vi "Assign Pixel to Wing Sector (FPGA).vi"(4 "End of Data?":bool, 6 "Valid Data?":bool, 7 "Pixel Intensity In":u8, 8 "Right Wing?":bool, 9 "Sector Parameters":T1, 10 "Pixel Y":u16, 11 "Pixel X":u16) -> (0 "Y Pixel Out":u16, 1 "Pixel Intensity Out":u8, 2 "sector #":u8, 3 "output valid":bool, 5 "X Pixel Out":u16)   [LabVIEW 2013]
uses:
  Sector Parameter Cluster.ctl
  <vilib>/rvi/FXPMathLib/FxpRectToPolar/subVIs/nifxpmath_RectToPolar_SimConfig.ctl
  <vilib>/rvi/FXPMathLib/FxpDiv/subVIs/nifxpmath_Div_SimConfig.ctl
  <vilib>/rvi/FXPMathLib/FxpRectToPolar/simVIs/DllFxpRectToPolarTemp_sub.vi
  <vilib>/rvi/FXPMathLib/FxpDiv/simVIs/DllFxpDivTemp_sub.vi
  <vilib>/rvi/FXPMathLib/FxpSub/XNode/nifxpmath_Sub.xnode
  <vilib>/rvi/FXPMathLib/FxpRectToPolar/XNode/nifxpmath_RectToPolar.xnode
  <vilib>/rvi/FXPMathLib/FxpAdd/XNode/nifxpmath_Add.xnode
  <vilib>/rvi/FXPMathLib/FxpDiv/XNode/nifxpmath_Div.xnode
  <vilib>/rvi/FXPMathLib/sim/FxpSim.dll
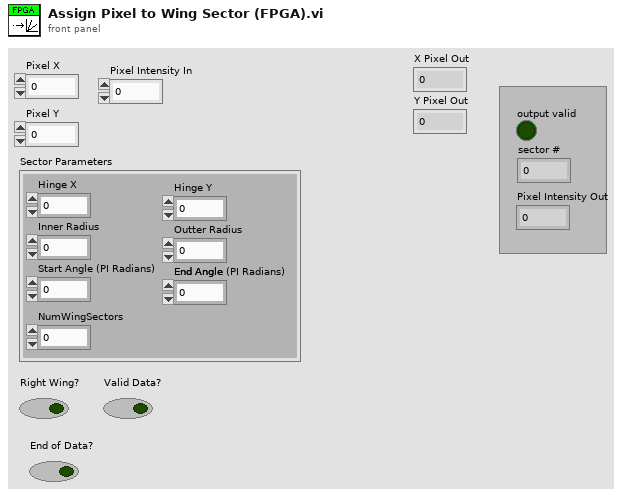
[diagram p1: front panel]
types:
  T1 = typedef "Sector Parameter Cluster.ctl" = cluster{"Start Angle":fxp<+/-,17,2>, "End Angle":fxp<+,17,3>, "Inner Radius":u16, "Outter Radius":u16, "Hinge X":u16, "Hinge Y":u16, "NumWingSectors":u8}
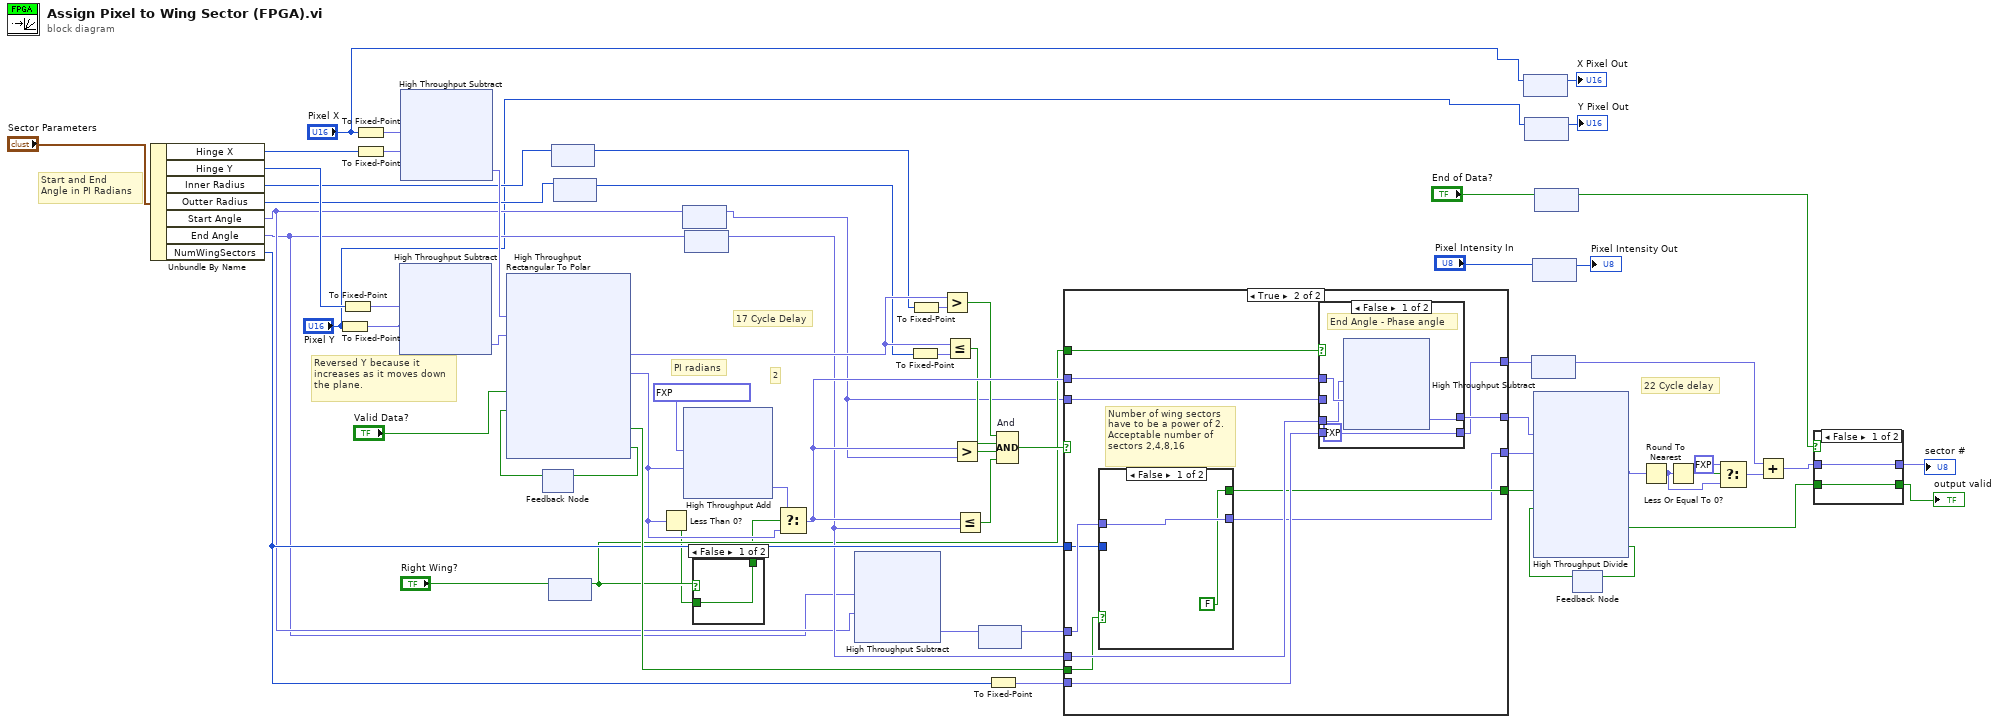
[diagram p0: block diagram]
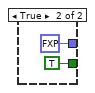
[diagram p2: hidden frame]
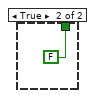
[diagram p3: hidden frame]
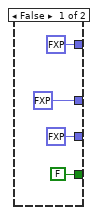
[diagram p4: hidden frame]
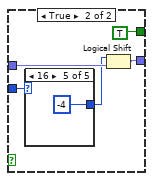
[diagram p5: hidden frame]
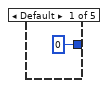
[diagram p6: hidden frame]
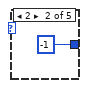
[diagram p7: hidden frame]
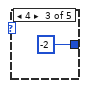
[diagram p8: hidden frame]
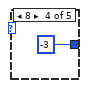
[diagram p9: hidden frame]
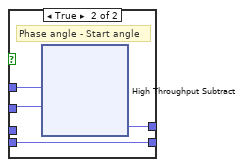
[diagram p10: hidden frame]
diagram:
  # "17 Cycle Delay"
  # "Reversed Y because it\nincreases as it moves down\nthe plane."
  # "PI radians"
  # "22 Cycle delay"
  # "Start and End\nAngle in PI Radians"
  # "2"
  n1 = Unbundle By Name("Sector Parameters") -> ("Hinge X"=w34:u16, "Hinge Y"=w51:u16, "Inner Radius"=w32:u16, "Outter Radius"=w30:u16, "Start Angle"=w16:fxp<+/-,17,2>, "End Angle"=w14:fxp<+,17,3>, "NumWingSectors"=w37:u8)
  n2 = To Fixed-Point(number="Pixel Y") -> (fixed-point=w41:fxp<+,11,11>)  [unwired: 1 in]
  n3 = To Fixed-Point(number=w51) -> (fixed-point=w42:fxp<+,11,11>)  [unwired: 1 in]
  n4 = To Fixed-Point(number="Pixel X") -> (fixed-point=w40:fxp<+,11,11>)  [unwired: 1 in]
  n5 = To Fixed-Point(number=w34) -> (fixed-point=w39:fxp<+,11,11>)  [unwired: 1 in]
  n6 = xnode "High Throughput Subtract"("x"=w42, "y"=w41) -> ("x-y"=w50:fxp<+/-,12,12>)
  n7 = xnode "High Throughput Subtract"("x"=w40, "y"=w39) -> ("x-y"=w49:fxp<+/-,12,12>)
  n8 = feedback #1() -> (w56:bool)  [unwired: 1 in]
  n9 = xnode "High Throughput Rectangular To Polar"("x"=w49, "y"=w50, "input valid"="Valid Data?", "ready for output (T)"=w56) -> ("magnitude"=w64:fxp<+,12,12>, "phase (pi)"=w61:fxp<+/-,16,2>, "output valid"=w38:bool, "ready for input"=w57:bool)
  n10 = feedback-in #1(w57) -> ()
  n11 = feedback #2() -> (w26:bool)  [unwired: 1 in]
  n12 = feedback-in #2("Right Wing?") -> ()
  n13 = feedback #3() -> (w31:u16)  [unwired: 1 in]
  n14 = feedback-in #3(w32) -> ()
  n15 = feedback #4() -> (w29:u16)  [unwired: 1 in]
  n16 = feedback-in #4(w30) -> ()
  n17 = Less Than 0?(x=w61) -> (x < 0?=w24:bool)
  n18 = feedback #5() -> (w15:fxp<+/-,17,2>)  [unwired: 1 in]
  n19 = feedback-in #5(w16) -> ()
  n20 = xnode ("High Throughput Add")("x"=fxp<+/-,16,2> 1.99993896484375 ("y"), "y"=w61) -> ("x+y"=w60:fxp<+/-,17,3>)
  n21 = feedback #6() -> (w28:fxp<+,17,3>)  [unwired: 1 in]
  n22 = feedback-in #6(w14) -> ()
  n23 = case shown="False" w26 {
    tunnel: [w66 FALSE ("s")] -> w25
    tunnel: w24 -> [w66 _]
    frame False {
    }
    frame True {
    }
  }
  n24 = Select(t=w60, s=w25, f=w61) -> (s? t:f=w58:fxp<+/-,17,3>)
  n25 = xnode ("High Throughput Subtract")("x"=w14, "y"=w16) -> ("x-y"=w13:fxp<+/-,17,6>)
  n26 = To Fixed-Point(number=w29) -> (fixed-point=w63:fxp<+,16,16>)  [unwired: 1 in]
  n27 = To Fixed-Point(number=w31) -> (fixed-point=w65:fxp<+,16,16>)  [unwired: 1 in]
  n28 = Greater?(x=w64, y=w65) -> (0:w55:bool)
  n29 = Less Or Equal?(x=w64, y=w63) -> (x <= y?=w54:bool)
  n30 = Greater?(x=w58, y=w15) -> (0:w53:bool)
  n31 = Less Or Equal?(x=w58, y=w28) -> (x <= y?=w52:bool)
  n32 = feedback #7() -> (w12:fxp<+/-,17,6>)  [unwired: 1 in]
  n33 = feedback-in #7(w13) -> ()
  n34 = To Fixed-Point(number=w37) -> (fixed-point=w22:fxp<+,8,8>)  [unwired: 1 in]
  n35 = Compound Arithmetic op=AND "And"(w55, w54, w53, w52) -> (w62:bool)
  n36 = case shown="True" w62 {
    tunnel: w58 -> [_ w83]
    tunnel: w15 -> [_ w82]
    tunnel: [fxp<+/-,17,6> 0.0 ("x-y") w73] -> w46
    tunnel: w28 -> [_ w80]
    tunnel: w22 -> [_ w81]
    tunnel: [fxp<+/-,20,5> 0.0 ("x-y") w79] -> w47
    tunnel: [FALSE ("output valid") w74] -> w45
    tunnel: [fxp<+,8,8> 0.0 w78] -> w43
    tunnel: w12 -> [_ w77]
    tunnel: w38 -> [_ w76]
    tunnel: w37 -> [_ w75]
    tunnel: w26 -> [_ w72]
    frame False {
    }
    frame True {
      # "Number of wing sectors\nhave to be a power of 2.\nAcceptable number of\nsectors 2,4,8,16"
      n37 = case shown="False" w76 {
        tunnel: w75 -> [_ w90]
        tunnel: w77 -> [w85 w89]
        tunnel: [w85 w87] -> w73
        tunnel: [FALSE ("output valid") TRUE ("output valid")] -> w74
        frame False {
        }
        frame True {
          n38 = case shown="16" w90 {
            tunnel: [i16 0 ("y") i16 -1 ("y") i16 -2 ("y") i16 -3 ("y") i16 -4 ("y")] -> w88
            frame Default {
            }
            frame 2 {
            }
            frame 4 {
            }
            frame 8 {
            }
            frame 16 {
            }
          }
          n39 = Logical Shift(y=w88, x=w89) -> (x << y=w87:fxp<+/-,17,6>)
        }
      }
      n40 = case shown="False" w72 {
        tunnel: w83 -> [w98 w103]
        tunnel: w82 -> [_ w102]
        tunnel: [w99 w101] -> w79
        tunnel: w81 -> [_ w100]
        tunnel: [fxp<+,8,8> 0.0 w100] -> w78
        tunnel: w80 -> [w97 _]
        frame False {
          # "End Angle - Phase angle"
          n41 = xnode "High Throughput Subtract"("x"=w97, "y"=w98) -> ("x-y"=w99:fxp<+/-,19,5>)
        }
        frame True {
          # "Phase angle - Start angle"
          n42 = xnode ("High Throughput Subtract")("x"=w103, "y"=w102) -> ("x-y"=w101:fxp<+/-,19,4>)
        }
      }
    }
  }
  n43 = feedback #8() -> (→"X Pixel Out":u16)  [unwired: 1 in]
  n44 = feedback-in #8("Pixel X") -> ()
  n45 = feedback #9() -> (→"Y Pixel Out":u16)  [unwired: 1 in]
  n46 = feedback-in #9("Pixel Y") -> ()
  n47 = feedback #10() -> (w17:fxp<+,8,8>)  [unwired: 1 in]
  n48 = feedback-in #10(w43) -> ()
  n49 = feedback #11() -> (→"Pixel Intensity Out":u8)  [unwired: 1 in]
  n50 = feedback-in #11("Pixel Intensity In") -> ()
  n51 = feedback #12() -> (w9:bool)  [unwired: 1 in]
  n52 = feedback-in #12("End of Data?") -> ()
  n53 = feedback #13() -> (w44:bool)  [unwired: 1 in]
  n54 = xnode "High Throughput Divide"("x"=w47, "y"=w46, "input valid"=w45, "ready for output (T)"=w44) -> ("x/y"=w19:fxp<+/-,20,16>, "output valid"=w5:bool, "ready for input"=w48:bool)
  n55 = feedback-in #13(w48) -> ()
  n56 = Round To Nearest(number=w19) -> (nearest integer value=w18:fxp<+/-,17,17>)
  n57 = Less Or Equal To 0?(x=w18) -> (x <= 0?=w21:bool)
  n58 = Select(t=fxp<+/-,17,17> 1.0, s=w21, f=w18) -> (s? t:f=w27:fxp<+/-,17,17>)
  n59 = Add(x=w17, y=w27) -> (x+y=w7:fxp<+/-,17,17>)
  n60 = case shown="False" w9 {
    tunnel: [w105 fxp<+/-,17,17> 0.0] -> w8
    tunnel: w7 -> [w105 _]
    tunnel: [w104 TRUE ("output valid")] -> w6
    tunnel: w5 -> [w104 _]
    frame False {
    }
    frame True {
    }
  }
  "output valid" <- w6
  "sector #" <- w8
